vi "Ramp-Step.vi"(7 "Controls":T1={"Start Freq (MHz)"=0.0, "Stop Freq (MHz)"=0.0, " Step (MHz)"=201.0} {"Step (MHz)" format="%#_13g"}, 11 "error in (no error)":errorcluster) -> (6 "Ary size(s)":i32, 8 "Freq (ary)":dbl[](array[numeric]), 12 "I Points":i32, 15 "error out":errorcluster)   [LabVIEW 2018]
panel:
  out "x = y?":bool
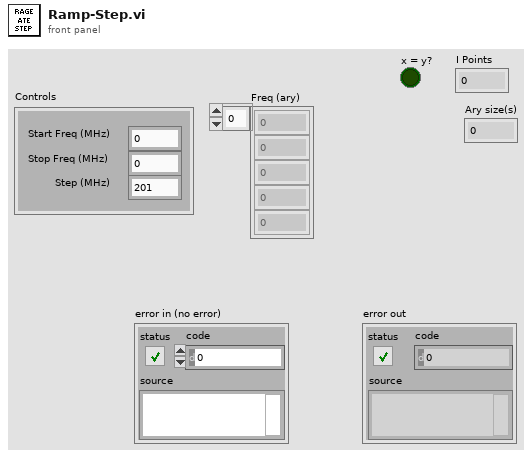
[diagram p1: front panel]
types:
  T1 = cluster{"Start Freq (MHz)":dbl, "Stop Freq (MHz)":dbl, " Step (MHz)":dbl}
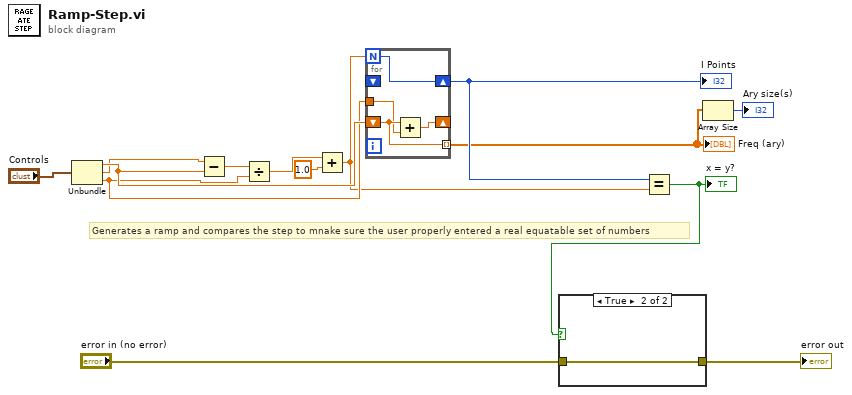
[diagram p0: block diagram]
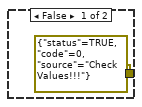
[diagram p2: hidden frame]
diagram:
  # "Generates a ramp and compares the step to mnake sure the user properly entered a real equatable set of numbers"
  n1 = Unbundle("Controls") -> ("Start Freq (MHz)"=w13:dbl, "Stop Freq (MHz)"=w12:dbl, "Step (MHz)"=w11:dbl)
  n2 = Subtract(x=w12, y=w13) -> (x-y=w9:dbl)
  n3 = Divide(x=w9, y=w11) -> (x/y=w8:dbl)
  n4 = Add(x=w8, y=1.0) -> (x+y=w6:dbl)
  n5 = for {
    N: w6 -> [w15]
    shift-right: [w17] -> _
    shift-left: w13 -> [w18]
    tunnel: [w18] -> w2 mode=indexing
    tunnel: w11 -> [w16]
    shift-right: [w15] -> w14
    shift-left: _ -> [_]
    n6 = Add(x=w18, y=w16) -> (x+y=w17:dbl)
  }
  "Freq (ary)" <- w2
  "I Points" <- w14
  n7 = Equal?(x=w14, y=w6) -> (x = y?=w3:bool)
  "x = y?" <- w3
  n8 = case shown="True" w3 {
    tunnel: "error in (no error)" -> [_ w20]
    tunnel: [errorcluster {"status"=TRUE, "code"=0, "source"="Check Values!!!"} ("error in (no error)") w20] -> w4
    frame False {
    }
    frame True {
    }
  }
  "error out" <- w4
  n9 = Array Size(array=w2) -> (size(s)=→"Ary size(s)":i32)
